vi "Tree Read Value.vi"(8 "error in (no error)":errorcluster, 11 "Tree Ref (generic)":refnum<vi>) -> (0 "error out":errorcluster, 2 "Value":string[](array[string]), 3 "Tree Ref (generic)":refnum<vi>)   [LabVIEW 2020, in "BetterDragAndDrop.lvlib" / "BetterTreeHandle.lvclass"]
uses:
  BetterTreeHandle.lvclass
  <vilib>/Utility/error.llb/Error Cluster From Error Code.vi
  <vilib>/ErrorRing/Error Ring.xnode
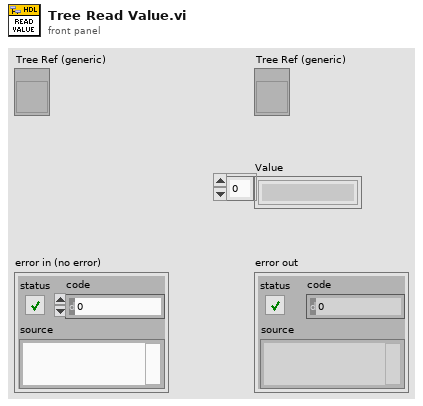
[diagram p1: front panel]
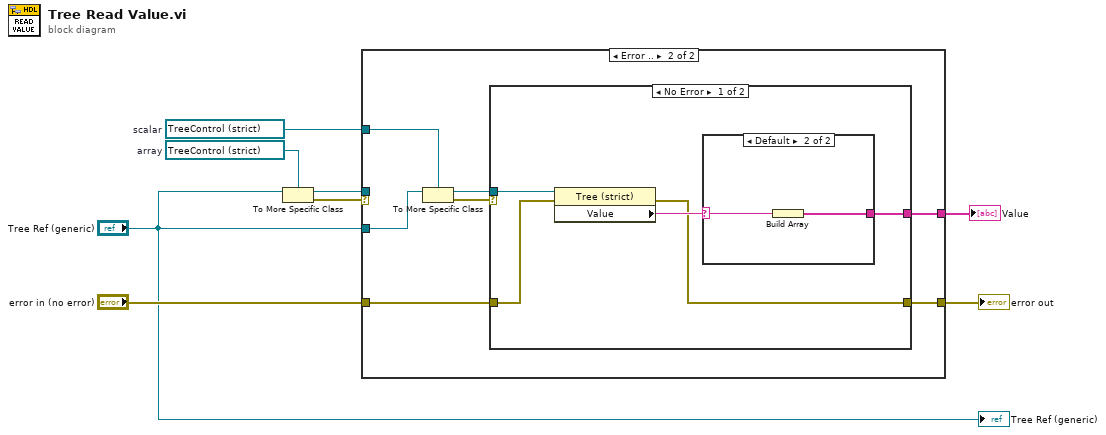
[diagram p0: block diagram]
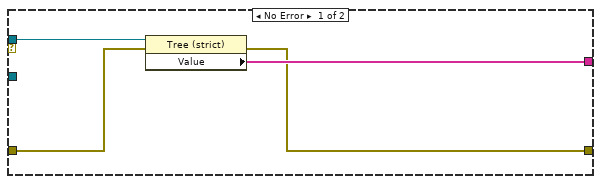
[diagram p2: hidden frame]
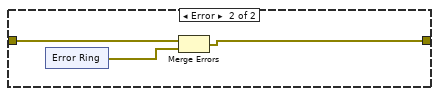
[diagram p4: hidden frame]
diagram:
  w4 = refnum<vi> refnum  # array
  w3 = refnum<vi> refnum  # scalar
  n1 = To More Specific Class(target class=w4, reference="Tree Ref (generic)") -> (specific class reference=w7:refnum<vi>, error out=w8:errorcluster)  [unwired: 1 in]
  n2 = case shown="Error .." w8 {
    tunnel: w7 -> [w12 _]
    tunnel: "Tree Ref (generic)" -> [_ w19]
    tunnel: w3 -> [_ w18]
    tunnel: "error in (no error)" -> [w10 w15]
    tunnel: [w9 w14] -> w5
    tunnel: [w11 w13] -> w1
    frame No Error {
      n3 = property class="Tree (strict)"(reference=w12, error in=w10) -> (error out=w9:errorcluster, "Value"=w11:string[])  [unwired: 1 out]
    }
    frame Error {
      n4 = To More Specific Class(target class=w18, reference=w19) -> (specific class reference=w16:refnum<vi>, error out=w17:errorcluster)  [unwired: 1 in]
      n5 = case shown="No Error" w17 {
        tunnel: w16 -> [w24 _]
        tunnel: w15 -> [w21 w28]
        tunnel: [w20 w27] -> w14
        tunnel: [w22 _] -> w13
        frame No Error {
          n6 = property class="Tree (strict)"(reference=w24, error in=w21) -> (error out=w20:errorcluster, "Value"=w23:string)  [unwired: 1 out]
          n7 = case shown="Default" w23 {
            selector: w23 -> [_ w26]
            tunnel: [_ w25] -> w22
            frame "" {
            }
            frame Default {
              n8 = Build Array(w26) -> (w25:string[])
            }
          }
        }
        frame Error {
          n9 = xnode "Error Ring"() -> ("error out"=w29:errorcluster)
          n10 = Merge Errors(w28, w29) -> (w27:errorcluster)
        }
      }
    }
  }
  "error out" <- w5
  "Value" <- w1
  "Tree Ref (generic)" <- "Tree Ref (generic)"
